vi "Ref plot window interface.vi"(6 "Bring to front (F)":bool, 8 "error in (no error)":errorcluster, 11 "Function":T1(ring)) -> (0 "error out":errorcluster, 3 "Ref plots window queue":refnum<queue>)   [LabVIEW 2017]
uses:
  Typedefs/HW config states enum.ctl
  Global Variables/General Globals.vi
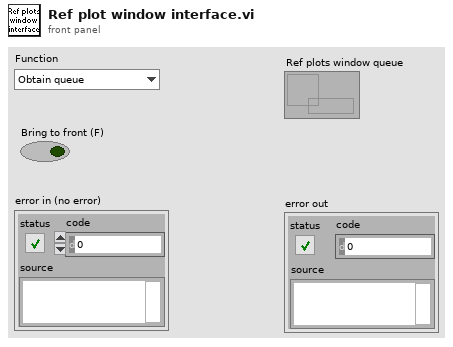
[diagram p1: front panel]
types:
  T1 = enum16{"Obtain queue", "Call window", "Call & send signal", "Release queue"}
  T2 = typedef "HW config states enum.ctl" = enum16{"Load from file", "Save to file", "Write all", "Read all", "Write XY stage settings", "Write DAQ FPGA settings", "Write Control FPGA settings", "Write Phys Channels", "Clear", "Compare from file"}
  T3 = typedef "Hardware Configuration settings.ctl" = cluster{"Computer MAC address":string, "XY Stage":T4, "Cam VidRec":T5, "Control Sys. HW config":T6, "DAQ FPGA HW Config":cluster{"Target":T7, "input card type":T8}, "DAQmx Chan":T9, "Encoder":T10, "Z Stage config cluster":T11, "Trigger HW config":T12, "Externalise Triggers":bool, "MC Supported":bool, "Laser 1 config cluster":T13, "Prechirper 1 config cluster":T14, "Laser Power Control HW config":T15, "No of AOD":u8, "Dev. PC":bool, "Swap XY on stage":bool, "Axial MC":bool}
  T4 = typedef "XY Stage config cluster.ctl" = cluster{"COM port":refnum<visa-resource-name>, "XY stage available":bool, "Baudrate":i32, "Type":string}
  T5 = typedef "Cam VidRec HW config setup cluster.ctl" = cluster{"DO flag-Video record":tag, "DO flag-Trial start":tag, "VidRec available":bool}
  T6 = typedef "Control Sys HW config cluster.ctl" = cluster{"Control system.FPGA available?":bool, "Control system.FPGA Type":string, "Control system.Network adapter name":string, "Control system.MAC address":string, "Control system.Ethernet Port":u32}
  T7 = typedef "nirio_resource_hc.ctl" = tag
  T8 = typedef "FPGA input type AC-DC.ctl" = enum16{"AC Card", "DC Card"}
  T9 = typedef "DAQmx physical channels cluster.ctl" = cluster{"Pockels AO":tag, "Hard shutter AO":tag, "PMT AOs":tag, "Power meter AI":tag}
  T10 = typedef "Encoder config cluster.ctl" = cluster{"IP address":string, "Port":u16, "Encoder available":bool, "Wheel radius (cm)":dbl, "Encoder Trigger":tag}
  T11 = typedef "Z Stage config cluster.ctl" = cluster{"COM port":refnum<visa-resource-name>, "Z stage available":bool, "Baudrate":i32, "Type":string}
  T12 = typedef "Triggers HW config.ctl" = cluster{"Available Device List":i32, "Device Address":string}
  T13 = typedef "Laser 1 config cluster.ctl" = cluster{"COM port":refnum<visa-resource-name>, "Laser 1 available":bool, "Baud Rate":i32, "Type":string}
  T14 = typedef "PreChirper 1 config cluster.ctl" = cluster{"COM port":refnum<visa-resource-name>, "Prechirper 1 \navailable":bool, "Baud Rate":i32, "Type":string}
  T15 = typedef "Laser Power Control HW config.ctl" = cluster{"Laser Power Control":string, "Laser Power Modulation Control":string}
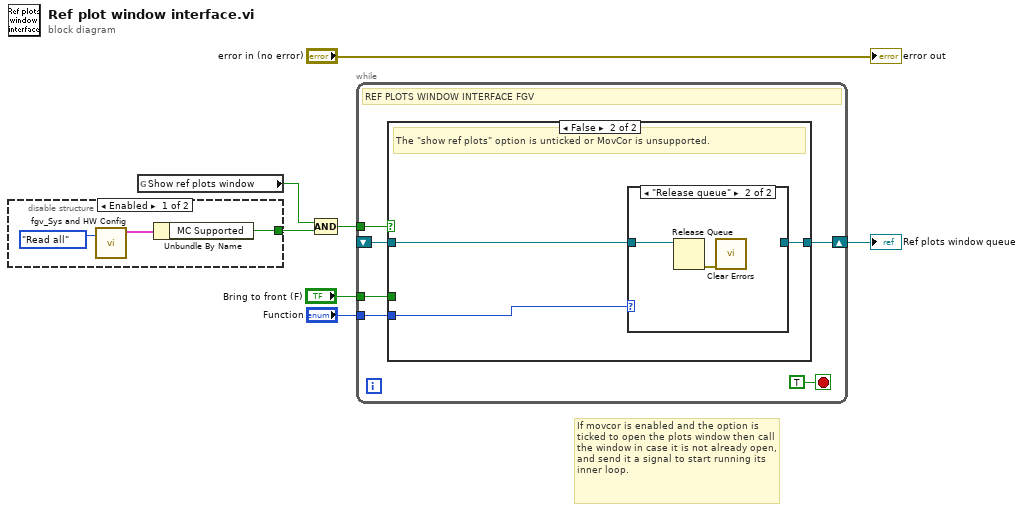
[diagram p0: block diagram]
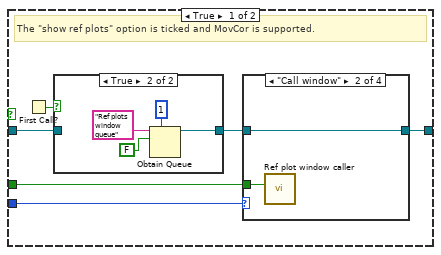
[diagram p2: hidden frame]
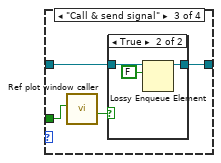
[diagram p5: hidden frame]
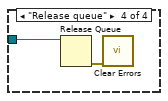
[diagram p7: hidden frame]
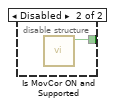
[diagram p9: hidden frame]
diagram:
  # "If movcor is enabled and the option is ticked to open the plots window then call the window in case it is not already open, and send it a signal to start running its inner loop."
  n1 = disable-structure shown="Enabled" {
    disable-tunnel: [w8 w11] -> w4
    frame Enabled {
      n2 = call "fgv_Sys and HW Config.vi"("Function"=HW_config_states_enum."Read all") -> ("Hardware Configuration OUT"=w10:T3)  [unwired: 8 in, 2 out]
      n3 = Unbundle By Name(w10) -> ("MC Supported"=w8:bool)
    }
    frame Disabled {
      n4 = call "Is MovCor ON and Supported.vi"() -> ("MovCor is ON and Supported"=w11:bool)  [unwired: 11 in]
    }
  }
  n5 = global read "General Globals.vi" "Show ref plots window"() -> (w5:bool)
  n6 = Compound Arithmetic op=AND(w5, w4) -> (w3:bool)
  n7 = while {
    shift-right: [w17] -> w6
    shift-left: _ -> [w16]
    tunnel: "Function" -> [w14]
    tunnel: w3 -> [w13]
    tunnel: "Bring to front (F)" -> [w12]
    stop <- TRUE stop-if-true
    # "REF PLOTS WINDOW INTERFACE FGV"
    n8 = case shown="False" w13 {
      tunnel: [w21 w44] -> w17
      tunnel: w16 -> [w20 w42]
      tunnel: w14 -> [w19 w43]
      tunnel: w12 -> [w18 _]
      frame True {
        # "The \"show ref plots\" option is ticked and MovCor is supported."
        n9 = First Call?() -> (First Call?: T/F=w23:bool)
        n10 = case shown="True" w23 {
          tunnel: [w24 w26] -> w22
          tunnel: w20 -> [w24 _]
          frame False {
          }
          frame True {
            n11 = Obtain Queue(max queue size (-1, unlimited)=1, name (unnamed)="Ref plots window queue", element data type=FALSE) -> (queue out=w26:refnum<queue>)  [unwired: 2 in, 2 out]
          }
        }
        n12 = case shown="\"Call window\"" w19 {
          tunnel: w22 -> [w29 w31 w34 w41]
          tunnel: [w29 w31 w33 _] -> w21
          tunnel: w18 -> [_ w30 w32 _]
          frame "Obtain queue", Default {
          }
          frame "Call window" {
            n13 = call "Ref plot window caller.vi"("Bring to front (F)"=w30) -> ()  [unwired: 10 in, 1 out]
          }
          frame "Call & send signal" {
            n14 = call "Ref plot window caller.vi"("Bring to front (F)"=w32) -> ("Window is open"=w35:bool)  [unwired: 10 in]
            n15 = case shown="True" w35 {
              tunnel: w34 -> [w36 w39]
              tunnel: [w36 w38] -> w33
              frame False {
              }
              frame True {
                n16 = Lossy Enqueue Element(queue=w39, element=FALSE) -> (queue out=w38:refnum<queue>)  [unwired: 1 in, 3 out]
              }
            }
          }
          frame "Release queue" {
            n17 = Release Queue(queue=w41) -> (error out=w40:errorcluster)  [unwired: 2 in, 2 out]
            n18 = call <vilib>:"Clear Errors.vi"("error in (no error)"=w40) -> ()  [unwired: 5 in, 2 out]
          }
        }
      }
      frame False {
        # "The \"show ref plots\" option is unticked or MovCor is unsupported."
        n19 = case shown="\"Release queue\"" w43 {
          tunnel: w42 -> [w45 w47]
          tunnel: [w45 _] -> w44
          frame Default {
          }
          frame "Release queue" {
            n20 = Release Queue(queue=w47) -> (error out=w46:errorcluster)  [unwired: 2 in, 2 out]
            n21 = call <vilib>:"Clear Errors.vi"("error in (no error)"=w46) -> ()  [unwired: 5 in, 2 out]
          }
        }
      }
    }
  }
  "Ref plots window queue" <- w6
  "error out" <- "error in (no error)"
